vi "Get Frequency and Amplitude.vi"(9 "Array in":dbl[](array[numeric]), 10 "df":dbl, 11 "f0":dbl) -> (1 "Array out":dbl[](array[numeric]), 2 "Frequency":dbl, 3 "Amplitude":dbl)   [LabVIEW 2014, in "Aquisicao de Dados.lvlib"]
uses:
  Aquisicao de Dados.lvlib
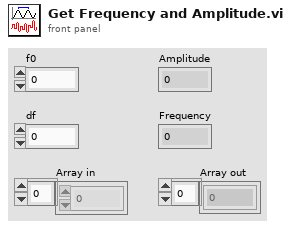
[diagram p1: front panel]
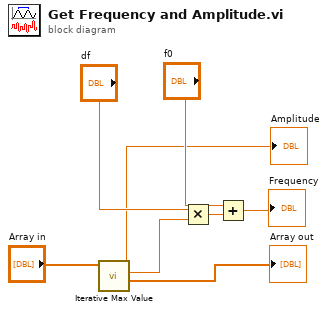
[diagram p0: block diagram]
diagram:
  n1 = call "Iterative Max Value.vi"("Array in"="Array in") -> ("Array out"=→"Array out":dbl[], "Max index"=w3:dbl, "Max value"=→"Amplitude":dbl)  [unwired: 8 in]
  n2 = Multiply(x="df", y=w3) -> (x*y=w2:dbl)
  n3 = Add(x="f0", y=w2) -> (x+y=→"Frequency":dbl)
